vi "Analise Taylor 1.vi"() -> ()   [LabVIEW 2013]
uses:
  <vilib>/Analysis/_algsub.llb/Vector Norm Type.ctl
  <vilib>/Analysis/_algsub.llb/Real Vector Norm.vi
  <vilib>/Waveform/WDTOps.llb/WDT Get Waveform Subset DBL.vi
  <vilib>/measure/NI_MAPro.lvlib
  <vilib>/Analysis/NI_AALPro.lvlib
panel:
  out "Frequencia Real":cluster{"Numeric":dbl}(graph)
  out "Amplitude Real":cluster{"Numeric":dbl}(graph)
  out "Fase Real (°)":cluster{"Numeric":dbl}(graph)
  out "resto(amostra)":dbl
  out "resto rad":dbl
  out "resto (segundos)":dbl
  out "Erro de Fase (°)":cluster{dbl}(graph)
  out "Fase Taylor 1 (rad)":dbl
  out "Fase":cluster{"Numeric":dbl, dbl}(graph)
  out "f0 real":dbl
  out "norm":dbl
  out "FE Real":dbl
  in  "SREAL Taylor 1 - v0 v1 f0 f1 p 2":dbl[](array[numeric])=[1.0, -0.33, 60.0, 0.1, 1.5707]
  out "Sinal Real normalizado":dbl[](graph)
  in  "t0":timestamp
  in  "dt":dbl
  out "best Sinal Real":dbl[](array[numeric])
  out "number":dbl[](array[numeric]) format="%_6e"
  in  "file (use dialog)":path=path "C:/Documents and Settings/mbmartins/Desktop/artigo ICHQP Belo Horizonte/Labview/VTENSAO.txt"
  out "nT":dbl format="%#.6p"
  out "x0 Taylor 1":dbl
  out "Amplitude Error":cluster{dbl, "y":dbl}(graph)
  out "n":i32
  out "T":dbl
  out "Amplitude":cluster{"Numeric":dbl, dbl}(graph)
  out "X(nT)":dbl
  out "amostras/janela":dbl
  out "Inicio janela":dbl
  out "Freq Error":cluster{dbl, dbl}(graph)
  out "Frequencia":cluster{"Numeric":dbl, dbl}(graph)
  out "sin(2pifnT - pi)":dbl
  in  "Fs report":i32=60
  out "timestamp":i32
  out "F(nT)":dbl format="%.6f"
  in  "Ciclos/janela":i32=3
  out "Fs (Hz)":dbl=5000.0 format="%#_12g"
  out "N amostras / ciclo":dbl
  out "T portadora":dbl=50.0 format="%0.1p"
  out "tempo total":dbl
  out "N amostras total":dbl
  in  "Ciclos total":i32=11
  in  "start/duration format":u16(ring) items=["Samples", "Relative Time"]
  in  "phase (rad)":dbl min=0.0 max=6.3 step=0.1
  in  "offset":dbl format="%0.2p"
  out "Frequency Taylor1":dbl format="%#_8f"
  out "best fit Taylor 1":dbl[](array[numeric])
  in  "Taylor 1 - v0 v1 f0 f1 p":dbl[](array[numeric])=[1.0, -0.33, 60.0, 0.1, 1.5707]
  in  "milliseconds to wait":u32
  out "FE Taylor 1":dbl
  out "Sinal de entrada (simulação)":string
  in  "fPM (Hz) deve ser igual fAM":dbl=1.0 min=0.0 max=2.0 step=0.1
  in  "fAm (Hz)":dbl=1.0 min=0.0 max=2.0 step=0.1
  in  "ka (PM)":dbl min=0.0 max=0.1 step=0.01
  in  "kx (AM)":dbl=0.1 min=0.0 max=0.1 step=0.01
  in  "reset signal":bool
  in  "frequency portadora":dbl=60.0 format="%0.6p"
  in  "amplitude portadora":dbl=1.0 format="%0.2p"
  # "Leitura de dados do arquivo"
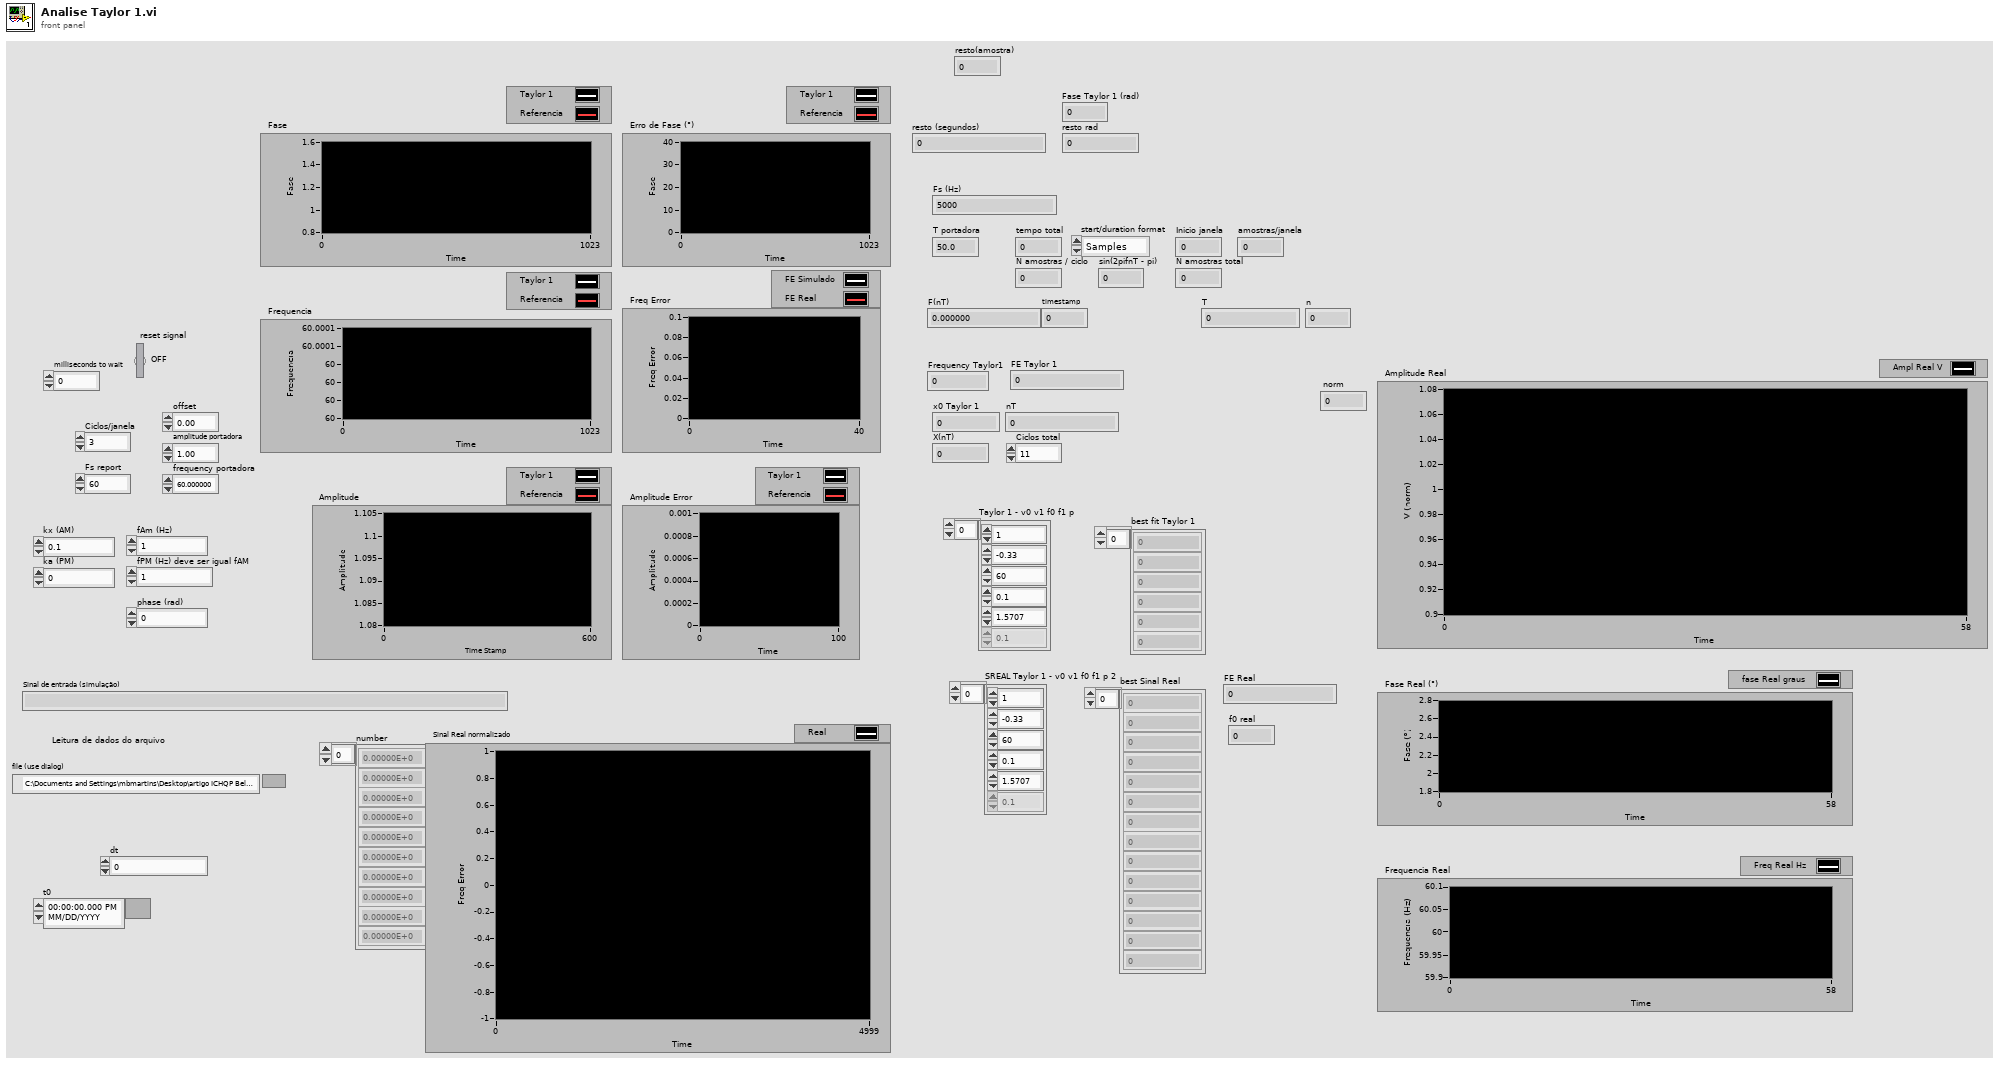
[diagram p1: front panel]
types:
  T1 = typedef "NI_AALPro.lvlib/Vector Norm Type.ctl" = u16
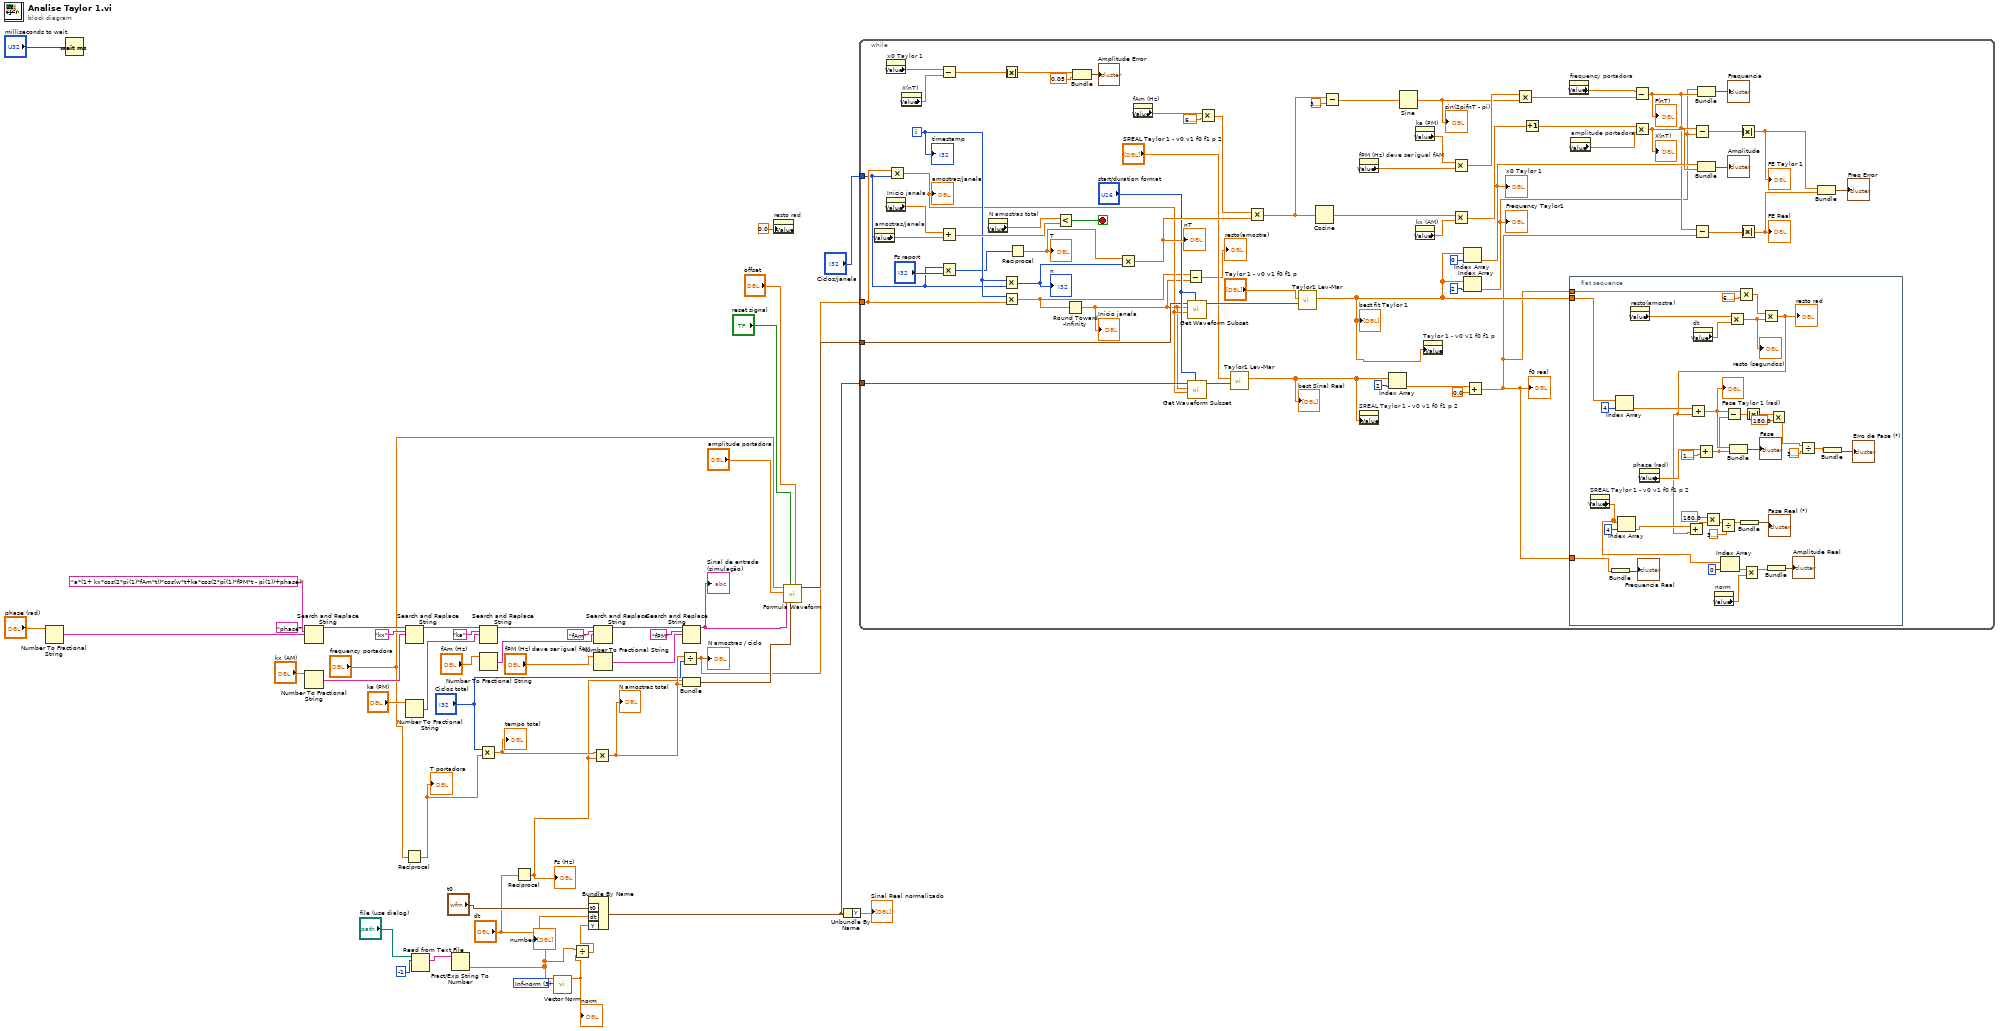
[diagram p0: block diagram]
diagram:
  w5 = T1 3 items=["1-norm"=1, "2-norm"=2, "Inf-norm"=3, "-Inf-norm"=4, "User Defined"=5] ("norm type")
  n1 = Number To Fractional String(number="phase (rad)") -> (F-format string=w25:string)  [unwired: 3 in]
  n2 = Wait (ms)(milliseconds to wait="milliseconds to wait") -> ()  [unwired: 1 out]
  n3 = Search and Replace String(input string="a*(1+ kx*cos(2*pi(1)*fAm*t))*cos(w*t+ka*cos(2*pi(1)*fPM*t - pi(1))+phase)" ("formula AM"), search string="phase", replace string=w25) -> (result string=w23:string)  [unwired: 5 in, 3 out]
  n4 = Number To Fractional String(number="kx (AM)") -> (F-format string=w43:string)  [unwired: 3 in]
  n5 = Search and Replace String(input string=w23, search string="kx", replace string=w43) -> (result string=w40:string)  [unwired: 5 in, 3 out]
  n6 = Number To Fractional String(number="ka (PM)") -> (F-format string=w37:string)  [unwired: 3 in]
  n7 = Reciprocal(x="frequency portadora") -> (1/x=w19:dbl)
  "T portadora" <- w19
  n8 = Read from Text File(file (use dialog)="file (use dialog)", count=-1) -> (text=w11:string[])  [unwired: 2 in, 3 out]
  n9 = Fract/Exp String To Number(string=w11) -> (number=w4:dbl[])  [unwired: 3 in, 1 out]
  "number" <- w4
  n10 = Multiply(x="Ciclos total", y=w19) -> (x*y=w20:dbl)
  "tempo total" <- w20
  n11 = Search and Replace String(input string=w40, search string="ka", replace string=w37) -> (result string=w39:string)  [unwired: 5 in, 3 out]
  n12 = Number To Fractional String(number="fAm (Hz)") -> (F-format string=w36:string)  [unwired: 3 in]
  n13 = Reciprocal(x="dt") -> (1/x=w10:dbl)
  "Fs (Hz)" <- w10
  n14 = call-poly <vilib>:"Vector Norm.vi"("norm type"=w5, "Input Vector"=w4) -> ("norm"=w3:dbl)  [unwired: 8 in, 1 out]
  "norm" <- w3
  n15 = Divide(x=w4, y=w3) -> (x/y=w2:dbl[])
  n16 = Bundle By Name("t0"="t0", "dt"="dt", "Y"=w2) -> (w7:waveform(dbl))  [unwired: 1 in]
  n17 = Multiply(x=w20, y=w10) -> (x*y=w17:dbl)
  "N amostras total" <- w17
  n18 = Search and Replace String(input string=w39, search string="fAm", replace string=w36) -> (result string=w38:string)  [unwired: 5 in, 3 out]
  n19 = Number To Fractional String(number="fPM (Hz) deve ser igual fAM") -> (F-format string=w35:string)  [unwired: 3 in]
  n20 = Divide(x=w17, y="Ciclos total") -> (x/y=w14:dbl)
  "N amostras / ciclo" <- w14
  n21 = Search and Replace String(input string=w38, search string="fPM", replace string=w35) -> (result string=w31:string)  [unwired: 5 in, 3 out]
  "Sinal de entrada (simulação)" <- w31
  n22 = Bundle(w10, w17) -> (w18:cluster{dbl, dbl})  [unwired: 1 in]
  n23 = property on="resto rad" class="DigNum (strict)"("Value"=0.0 ("resto rad")) -> ()  [unwired: 2 in, 2 out]
  n24 = call <vilib>:"Formula Waveform.vi"("offset"="offset", "sampling info"=w18, "reset signal"="reset signal", "formula"=w31, "amplitude"="amplitude portadora", "frequency"="frequency portadora") -> ("signal out"=w22:waveform(dbl))  [unwired: 4 in, 1 out]
  n25 = Unbundle By Name(w7) -> ("Y"=→"Sinal Real normalizado":dbl[])
  n26 = while {
    tunnel: w22 -> [w63]
    tunnel: w14 -> [w110]
    tunnel: "Ciclos/janela" -> [w88]
    tunnel: w7 -> [w64]
    i -> [w90]
    stop <- w94 stop-if-true
    n27 = property on="amostras/janela" class="DigNum (strict)"() -> ("Value"=w86:dbl)  [unwired: 2 in, 2 out]
    n28 = property on="x0 Taylor 1" class="DigNum (strict)"() -> ("Value"=w72:dbl)  [unwired: 2 in, 2 out]
    n29 = property on="Inicio janela" class="DigNum (strict)"() -> ("Value"=w93:dbl)  [unwired: 2 in, 2 out]
    n30 = Multiply(x=w110, y=w88) -> (x*y=w54:dbl)
    "amostras/janela" <- w54
    n31 = property on="X(nT)" class="DigNum (strict)"() -> ("Value"=w70:dbl)  [unwired: 2 in, 2 out]
    n32 = Subtract(x=w72, y=w70) -> (x-y=w73:dbl)
    n33 = Add(x=w93, y=w86) -> (x+y=w92:dbl)
    n34 = Multiply(x=w88, y="Fs report") -> (x*y=w89:i32)
    n35 = property on="N amostras total" class="DigNum (strict)"() -> ("Value"=w95:dbl)  [unwired: 2 in, 2 out]
    n36 = Absolute Value(x=w73) -> (abs(x)=w71:dbl)
    n37 = Multiply(x=w90, y=w88) -> (x*y=w91:i32)
    "n" <- w91
    n38 = Multiply(x=w90, y=w110) -> (x*y=w53:dbl)
    n39 = Reciprocal(x=w89) -> (1/x=w99:dbl)
    "T" <- w99
    n40 = Less?(x=w95, y=w92) -> (x < y?=w94:bool)
    n41 = Round Toward -Infinity(1:w53) -> (0:w52:dbl)
    "Inicio janela" <- w52
    n42 = Bundle(w71, "y"=0.05) -> (→"Amplitude Error":cluster{dbl, "y":dbl})  [unwired: 1 in]
    n43 = Multiply(x=w99, y=w91) -> (x*y=w104:dbl)
    "nT" <- w104
    n44 = property on="fAm (Hz)" class="DigNum (strict)"() -> ("Value"=w75:dbl)  [unwired: 2 in, 2 out]
    n45 = Subtract(x=w53, y=w52) -> (x-y=→"resto(amostra)":dbl)
    n46 = call-poly <vilib>:"Get Waveform Subset.vi"("start/duration format"="start/duration format", "duration"=w54, "start samples/time"=w52, "waveform in"=w63) -> ("waveform out"=w66:waveform(dbl))  [unwired: 2 in, 3 out]
    n47 = call-poly <vilib>:"Get Waveform Subset.vi"("start/duration format"="start/duration format", "duration"=w54, "start samples/time"=w52, "waveform in"=w64) -> ("waveform out"=w65:waveform(dbl))  [unwired: 2 in, 3 out]
    n48 = Multiply(x=w75, y=6.283185307179586) -> (x*y=w105:dbl)
    n49 = call "Taylor1 Lev-Mar.vi"("signal in"=w65, "initial parameters"="SREAL Taylor 1 - v0 v1 f0 f1 p 2") -> ("best fit parameters"=w56:dbl[])  [unwired: 5 in, 4 out]
    "best Sinal Real" <- w56
    n50 = Multiply(x=w105, y=w104) -> (x*y=w84:dbl)
    n51 = call "Taylor1 Lev-Mar.vi"("signal in"=w66, "initial parameters"="Taylor 1 - v0 v1 f0 f1 p") -> ("best fit parameters"=w49:dbl[])  [unwired: 5 in, 4 out]
    "best fit Taylor 1" <- w49
    n52 = Cosine(x=w84) -> (cos(x)=w83:dbl)
    n53 = Subtract(x=w84, y=3.141592653589793) -> (x-y=w87:dbl)
    n54 = property on="fPM (Hz) deve ser igual fAM" class="DigNum (strict)"() -> ("Value"=w106:dbl)  [unwired: 2 in, 2 out]
    n55 = property on="SREAL Taylor 1 - v0 v1 f0 f1 p 2" class="Arr (strict)"("Value"=w56) -> ()  [unwired: 2 in, 2 out]
    n56 = Index Array(array=w56, index=2) -> (element=w60:dbl)
    n57 = Sine(x=w87) -> (sin(x)=w101:dbl)
    "sin(2pifnT - pi)" <- w101
    n58 = property on="ka (PM)" class="DigNum (strict)"() -> ("Value"=w108:dbl)  [unwired: 2 in, 2 out]
    n59 = property on="kx (AM)" class="DigNum (strict)"() -> ("Value"=w85:dbl)  [unwired: 2 in, 2 out]
    n60 = property on="Taylor 1 - v0 v1 f0 f1 p" class="Arr (strict)"("Value"=w49) -> ()  [unwired: 2 in, 2 out]
    n61 = Multiply(x=w108, y=w106) -> (x*y=w102:dbl)
    n62 = Multiply(x=w83, y=w85) -> (x*y=w82:dbl)
    n63 = Index Array(array=w49, index=0) -> (element=w77:dbl)
    "x0 Taylor 1" <- w77
    n64 = Index Array(array=w49, index=2) -> (element=w50:dbl)
    "Frequency Taylor1" <- w50
    n65 = Add(x=w60, y=0.0) -> (x+y=w48:dbl)
    "f0 real" <- w48
    n66 = Multiply(x=w102, y=w101) -> (x*y=w98:dbl)
    n67 = Increment(x=w82) -> (x+1=w81:dbl)
    n68 = property on="frequency portadora" class="DigNum (strict)"() -> ("Value"=w109:dbl)  [unwired: 2 in, 2 out]
    n69 = flat-sequence {
      tunnel: w49 -> [w149]
      tunnel: w48 -> [w136]
      tunnel: w48 -> [w120]
      frame #0 {
        n70 = property on="SREAL Taylor 1 - v0 v1 f0 f1 p 2" class="Arr (strict)"() -> ("Value"=w118:dbl[])  [unwired: 2 in, 2 out]
        n71 = Bundle(w120) -> (→"Frequencia Real":cluster{dbl})  [unwired: 1 in]
        n72 = Index Array(array=w149, index=4) -> (element=w138:dbl)
        n73 = Index Array(array=w118, index=4) -> (element=w132:dbl)
        n74 = property on="resto(amostra)" class="DigNum (strict)"() -> ("Value"=w137:dbl)  [unwired: 2 in, 2 out]
        n75 = property on="phase (rad)" class="DigNum (strict)"() -> ("Value"=w148:dbl)  [unwired: 2 in, 2 out]
        n76 = property on="dt" class="DigNum (strict)"() -> ("Value"=w143:dbl)  [unwired: 2 in, 2 out]
        n77 = Add(x=w148, y=1.5707963267948966) -> (x+y=w131:dbl)
        n78 = property on="norm" class="DigNum (strict)"() -> ("Value"=w114:dbl)  [unwired: 2 in, 2 out]
        n79 = Index Array(array=w118, index=0) -> (element=w117:dbl)
        n80 = Multiply(x=w137, y=w143) -> (x*y=w140:dbl)
        "resto (segundos)" <- w140
        n81 = Multiply(x=w136, y=6.283185307179586) -> (x*y=w141:dbl)
        n82 = Multiply(x=w117, y=w114) -> (x*y=w115:dbl)
        n83 = Multiply(x=w141, y=w140) -> (x*y=w130:dbl)
        "resto rad" <- w130
        n84 = Add(x=w132, y=w130) -> (x+y=w133:dbl)
        n85 = Add(x=w138, y=w130) -> (x+y=w139:dbl)
        "Fase Taylor 1 (rad)" <- w139
        n86 = Multiply(x=180.0, y=w133) -> (x*y=w125:dbl)
        n87 = Divide(x=w125, y=3.141592653589793) -> (x/y=w123:dbl)
        n88 = Subtract(x=w139, y=w131) -> (x-y=w146:dbl)
        n89 = Bundle(w139, w131) -> (→"Fase":cluster{dbl, dbl})  [unwired: 1 in]
        n90 = Bundle(w123) -> (→"Fase Real (°)":cluster{dbl})  [unwired: 1 in]
        n91 = Absolute Value(x=w146) -> (abs(x)=w144:dbl)
        n92 = Bundle(w115) -> (→"Amplitude Real":cluster{dbl})  [unwired: 1 in]
        n93 = Multiply(x=w144, y=180.0) -> (x*y=w127:dbl)
        n94 = Divide(x=w127, y=3.141592653589793) -> (x/y=w128:dbl)
        n95 = Bundle(w128) -> (→"Erro de Fase (°)":cluster{dbl})  [unwired: 1 in]
      }
    }
    n96 = property on="amplitude portadora" class="DigNum (strict)"() -> ("Value"=w80:dbl)  [unwired: 2 in, 2 out]
    n97 = Subtract(x=w109, y=w98) -> (x-y=w59:dbl)
    "F(nT)" <- w59
    n98 = Multiply(x=w81, y=w80) -> (x*y=w79:dbl)
    "X(nT)" <- w79
    n99 = Subtract(x=w59, y=w50) -> (x-y=w112:dbl)
    n100 = Subtract(x=w59, y=w48) -> (x-y=w58:dbl)
    n101 = Bundle("Numeric"=w50, w59) -> (→"Frequencia":cluster{"Numeric":dbl, dbl})  [unwired: 1 in]
    n102 = Bundle("Numeric"=w77, w79) -> (→"Amplitude":cluster{"Numeric":dbl, dbl})  [unwired: 1 in]
    n103 = Absolute Value(x=w112) -> (abs(x)=w113:dbl)
    "FE Taylor 1" <- w113
    n104 = Absolute Value(x=w58) -> (abs(x)=w57:dbl)
    "FE Real" <- w57
    n105 = Bundle(w113, w57) -> (→"Freq Error":cluster{dbl, dbl})  [unwired: 1 in]
    "timestamp" <- w90
  }
